vi "Error Query.vi"(8 "error in (no error)":errorcluster, 10 "VISA resource name":refnum<visa-resource-name>, 11 "Electrometer in":refnum<class "Electrometer.lvclass">) -> (0 "error out":errorcluster, 1 "Error Message":string, 2 "Error Code":i32[](array[numeric]), 3 "Electrometer out":refnum<class "Electrometer.lvclass">)   [LabVIEW 2016, in "Electrometer.lvclass"]
doc: "Queries the instrument for any errors in the instrument's error queue. It will continue to read errors until all errors have been read from the instrument. Any errors will be returned in the <B>error out</B> control.\n\n<B>Note:</B>\nThis VI is called automatically by most driver VIs so it is not usually necessary to call this in an application."
uses:
  Electrometer/Electrometer.lvclass
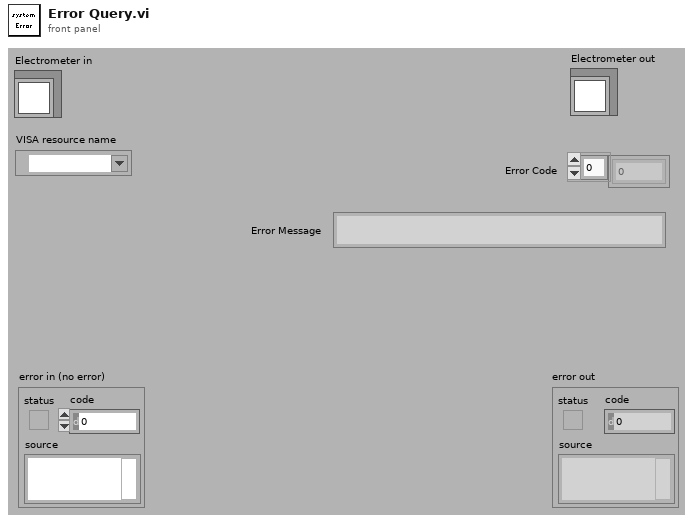
[diagram p1: front panel]
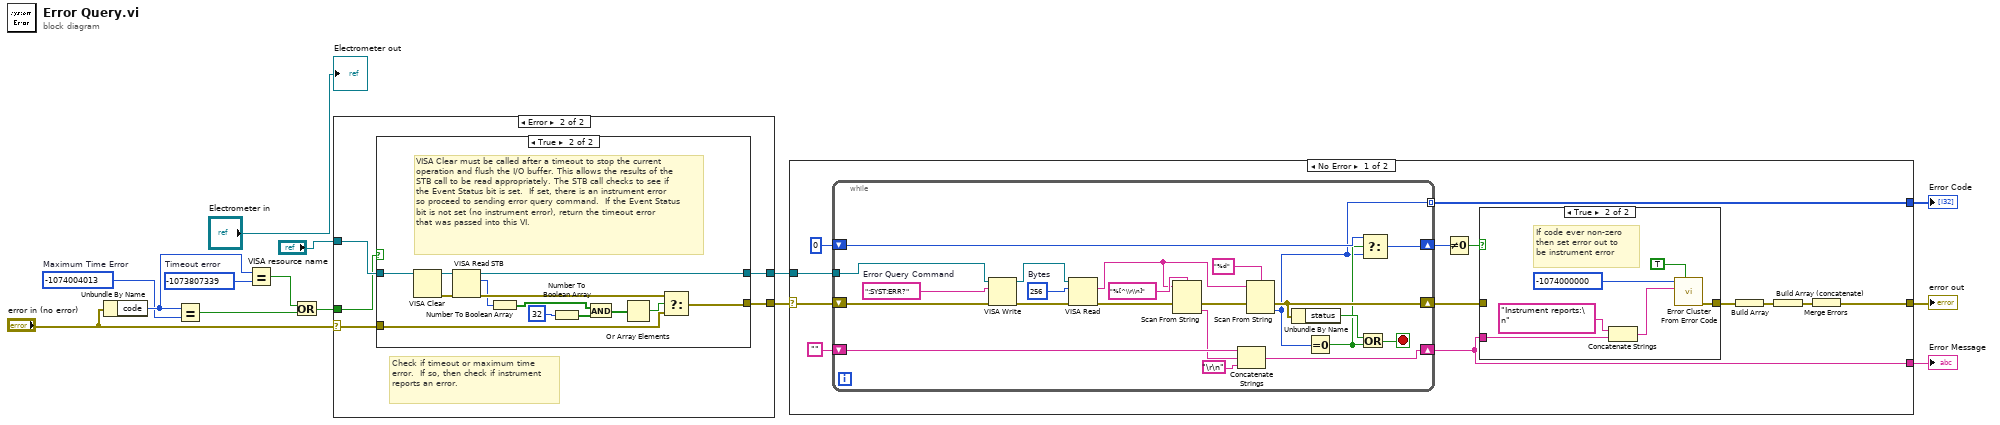
[diagram p0: block diagram]
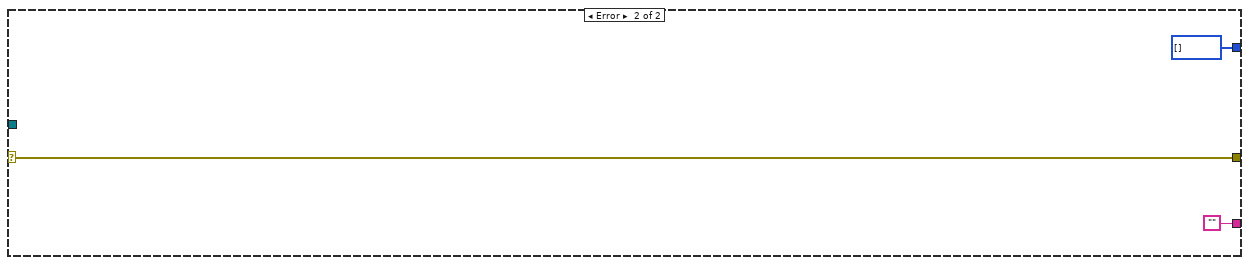
[diagram p5: hidden frame]
diagram:
  w7 = -1074004013  # Maximum Time Error
  w9 = -1073807339  # Timeout error
  n1 = Unbundle By Name("error in (no error)") -> ("code"=w8:i32)
  n2 = Equal?(x=w8, y=w7) -> (x = y?=w6:bool)
  n3 = Equal?(x=w8, y=w9) -> (x = y?=w5:bool)
  n4 = Or(x=w5, y=w6) -> (x .or. y?=w4:bool)
  n5 = case shown="Error" "error in (no error)" {
    selector: "error in (no error)" -> [w15 w19]
    tunnel: "VISA resource name" -> [w16 w21]
    tunnel: [w16 w20] -> w10
    tunnel: [w15 w18] -> w11
    tunnel: w4 -> [_ w17]
    frame No Error {
    }
    frame Error {
      # "Check if timeout or maximum time error.  If so, then check if instrument reports an error."
      n6 = case shown="True" w17 {
        tunnel: w21 -> [w23 w29]
        tunnel: [w23 w26] -> w20
        tunnel: w19 -> [w22 w32]
        tunnel: [w22 w31] -> w18
        frame False {
          # "Error code not a timeout, so best to pass on to user."
        }
        frame True {
          # "VISA Clear must be called after a timeout to stop the current operation and flush the I/O buffer. This allows the results of the  STB call to be read appropriately. The STB call checks to see if the Event Status bit is set.  If set, there is an instrument error so proceed to sending error query command.  If the Event Status bit is not set (no instrument error), return the timeout error that was passed into this VI."
          n7 = VISA Clear(VISA resource name=w29) -> (VISA resource name out=w28:refnum<visa-resource-name>, error out=w27:errorcluster)  [unwired: 1 in]
          n8 = VISA Read STB(8:w27, 11:w28) -> (0:w25:errorcluster, 2:w24:u16, 3:w26:refnum<visa-resource-name>)
          n9 = Number To Boolean Array(number=w24) -> (Boolean array=w33:bool[])
          n10 = Number To Boolean Array(number=32) -> (Boolean array=w35:bool[])
          n11 = And(x=w33, y=w35) -> (x .and. y?=w34:bool[])
          n12 = Or Array Elements(Boolean array=w34) -> (logical OR=w30:bool)
          n13 = Select(t=w25, s=w30, f=w32) -> (s? t:f=w31:errorcluster)
        }
      }
    }
  }
  n14 = case shown="No Error" w11 {
    selector: w11 -> [w39 w79]
    tunnel: w10 -> [w49 _]
    tunnel: [w47 w79] -> w14
    tunnel: [w42 ""] -> w13
    tunnel: [w41 i32[] []] -> w12
    frame No Error {
      n15 = while {
        tunnel: w49 -> [w78]
        shift-right: [w66] -> w42
        shift-left: "" -> [w69]
        shift-right: [w64] -> w43
        shift-left: 0 -> [w65]
        shift-right: [w62] -> w40
        shift-left: w39 -> [w63]
        tunnel: [w57] -> w41 mode=indexing
        stop <- w72 stop-if-true
        w76 = u32 256  # Bytes
        w74 = ":SYST:ERR?"  # Error Query Command
        n16 = VISA Write(VISA resource name=w78, write buffer=w74, error in (no error)=w63) -> (VISA resource name out=w77:refnum<visa-resource-name>, error out=w75:errorcluster)  [unwired: 1 out]
        n17 = VISA Read(VISA resource name=w77, byte count=w76, error in (no error)=w75) -> (read buffer=w70:string, error out=w61:errorcluster)  [unwired: 2 out]
        n18 = Scan From String(format string="%[^\\r\\n]", input string=w70, error in=w61) -> (error out=w60:errorcluster, output 1=w67:string)  [unwired: 2 in, 2 out]
        n19 = Concatenate Strings(w69, w67, "\r\n") -> (w66:string)
        n20 = Scan From String(format string="%d", input string=w70, error in=w60) -> (error out=w62:errorcluster, output 1=w57:i32)  [unwired: 2 in, 2 out]
        n21 = Unbundle By Name(w62) -> ("status"=w59:bool)
        n22 = Equal To 0?(x=w57) -> (x = 0?=w58:bool)
        n23 = Or(x=w59, y=w58) -> (x .or. y?=w72:bool)
        n24 = Select(t=w65, s=w58, f=w57) -> (s? t:f=w64:i32)
      }
      n25 = Not Equal To 0?(x=w43) -> (x != 0?=w45:bool)
      n26 = case shown="True" w45 {
        tunnel: w42 -> [_ w55]
        tunnel: [w50 w51] -> w44
        tunnel: w40 -> [w50 _]
        frame False {
        }
        frame True {
          # "If code ever non-zero\nthen set error out to\nbe instrument error"
          n27 = Concatenate Strings("Instrument reports:\n" ("Source"), w55) -> (w52:string)
          n28 = call <vilib>:"Error Cluster From Error Code.vi"("show call chain? (False)"=TRUE, "error message (\"\")"=w52, "error code (0)"=-1074000000 ("Code")) -> ("error out"=w51:errorcluster)  [unwired: 6 in]
        }
      }
      n29 = Build Array(w44) -> (w38:errorcluster[])
      n30 = Build Array (concatenate)(w38) -> (w37:errorcluster[])
      n31 = Merge Errors(w37) -> (w47:errorcluster)
    }
    frame Error {
    }
  }
  "error out" <- w14
  "Error Message" <- w13
  "Error Code" <- w12
  "Electrometer out" <- "Electrometer in"
